vi "Reduce Stock Level and Check.vi"(8 "error in (no error)":errorcluster, 10 "Product Index":i32, 11 "Data Cluster":T1) -> (0 "error out":errorcluster, 2 "Sucessful":bool, 3 "Data Cluster Out":T1)   [LabVIEW 2019, in "Stock.lvlib"]
uses:
  Stock.lvlib
  Module Data--cluster.ctl
  Products.ctl
  <vilib>/Utility/xml.llb/Write to XML File(string).vi
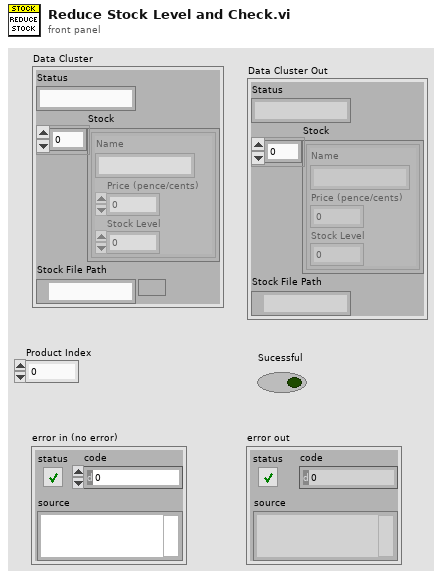
[diagram p1: front panel]
types:
  T1 = typedef "Stock.lvlib/Module Data--cluster.ctl" = cluster{"Status":string, "Stock":T2[], "Stock File Path":path}
  T2 = typedef "Stock.lvlib/Products.ctl" = cluster{"Name":string, "Price (pence/cents)":u32, "Stock Level":u32}
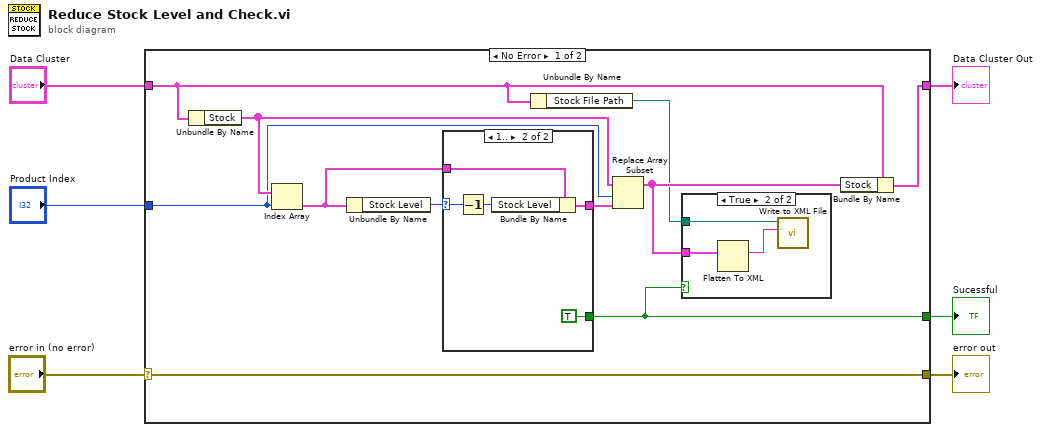
[diagram p0: block diagram]
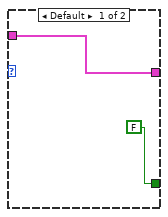
[diagram p3: hidden frame]
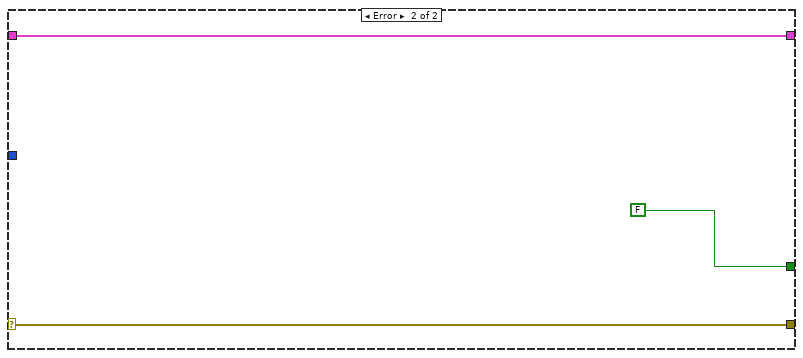
[diagram p4: hidden frame]
diagram:
  n1 = case shown="No Error" "error in (no error)" {
    selector: "error in (no error)" -> [w13 w28]
    tunnel: "Product Index" -> [w11 _]
    tunnel: "Data Cluster" -> [w8 w30]
    tunnel: [w14 w30] -> w4
    tunnel: [w10 FALSE] -> w3
    tunnel: [w13 w28] -> w1
    frame No Error {
      n2 = Unbundle By Name(w8) -> ("Stock"=w16:T2[])
      n3 = Index Array(array=w16, index=w11) -> (element=w17:T2)
      n4 = Unbundle By Name(w17) -> ("Stock Level"=w12:u32)
      n5 = case shown="1.." w12 {
        selector: w12 -> [_ w26]
        tunnel: [FALSE TRUE] -> w10
        tunnel: w17 -> [w21 w27]
        tunnel: [w21 w25] -> w15
        frame Default {
        }
        frame 1.. {
          n6 = Decrement(x=w26) -> (x-1=w23:u32)
          n7 = Bundle By Name(cluster=w27, "Stock Level"=w23) -> (w25:T2)
        }
      }
      n8 = Unbundle By Name(w8) -> ("Stock File Path"=w7:path)
      n9 = Replace Array Subset(array=w16, new element=w15, index=w11) -> (w9:T2[])
      n10 = case shown="True" w10 {
        tunnel: w9 -> [_ w19]
        tunnel: w7 -> [_ w20]
        frame False {
        }
        frame True {
          n11 = Flatten To XML(anything=w19) -> (xml string=w18:string)
          n12 = call-poly <vilib>:"Write to XML File.vi"("XML Input"=w18, "XML File Path"=w20) -> ()  [unwired: 7 in, 3 out]
        }
      }
      n13 = Bundle By Name(cluster=w8, "Stock"=w9) -> (w14:T1)
    }
    frame Error {
    }
  }
  "Data Cluster Out" <- w4
  "error out" <- w1
  "Sucessful" <- w3
